vi "Get Logout Path.vi"(8 "error in (no error)":errorcluster, 11 "SOL Auth in":refnum<class "SOL Auth.lvclass">) -> (0 "error out":errorcluster, 2 "Logout Path":string, 3 "SOL Auth out":refnum<class "SOL Auth.lvclass">)   [LabVIEW 2020, in "Summer of LabVIEW.lvlib" / "SOL Auth.lvclass"]
uses:
  SOL Auth.lvclass
  SOL Auth.lvclass/SOL Auth.ctl
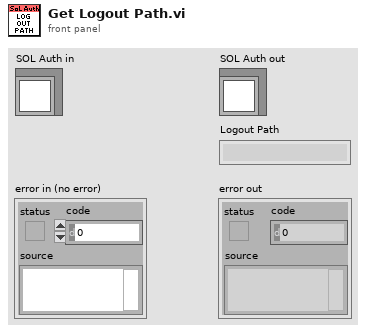
[diagram p1: front panel]
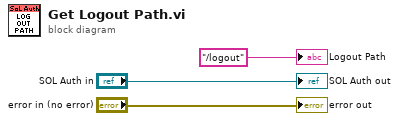
[diagram p0: block diagram]
diagram:
  "error out" <- "error in (no error)"
  "SOL Auth out" <- "SOL Auth in"
  "Logout Path" <- "/logout" ("Logout Path")
